vi "DllFxpAddSub_Fxp.vi"(6 "cin/nbin":bool, 8 "load":bool=TRUE, 9 "is sub":bool, 10 "y":fxp<+,32,32>, 11 "x":fxp<+,32,32>) -> (2 "cout/nbout/overflow":bool, 3 "s":fxp<+,32,32>)   [LabVIEW 2017]
uses:
  <vilib>/rvi/FXPMathLib/sim/FxpSim.dll
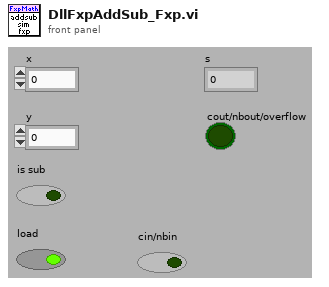
[diagram p1: front panel]
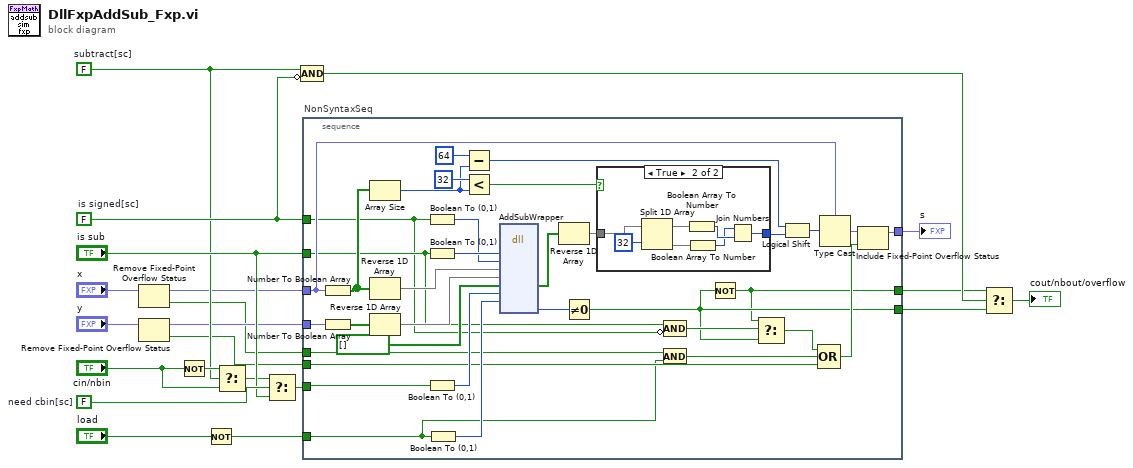
[diagram p0: block diagram]
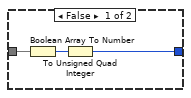
[diagram p2: hidden frame]
diagram:
  w11 = FALSE  # subtract[sc]
  w12 = FALSE  # is signed[sc]
  w21 = FALSE  # need cbin[sc]
  n1 = Remove Fixed-Point Overflow Status(3:"x") -> (0:w3:bool, 1:w6:fxp<+,32,32>)
  n2 = Remove Fixed-Point Overflow Status(3:"y") -> (0:w2:bool, 1:w4:fxp<+,32,32>)
  n3 = Not(x="cin/nbin") -> (.not. x?=w16:bool)
  n4 = Not(x="load") -> (.not. x?=w9:bool)
  n5 = Select(t=w16, s=w11, f="cin/nbin") -> (s? t:f=w17:bool)
  n6 = Select(t=w17, s=w21, f="is sub") -> (s? t:f=w20:bool)
  n7 = Compound Arithmetic op=AND(w11, invert w12) -> (w10:bool)
  n8 = stacked-sequence "NonSyntaxSeq" {
    tunnel: [w24] -> w14
    tunnel: "is sub" -> [w27]
    tunnel: w20 -> [w54]
    tunnel: w9 -> [w30]
    tunnel: w12 -> [w26]
    tunnel: w6 -> [w35]
    tunnel: w4 -> [w42]
    tunnel: [w33] -> w8
    tunnel: w3 -> [w29]
    tunnel: w2 -> [w31]
    tunnel: [w23] -> w1
    frame #0 {
      n9 = Number To Boolean Array(number=w35) -> (Boolean array=w43:bool[])
      n10 = Number To Boolean Array(number=w42) -> (Boolean array=w41:bool[])
      n11 = Array Size(array=w43) -> (size(s)=w40:i32)
      n12 = Reverse 1D Array(array=w43) -> (reversed array=w44:bool[])
      n13 = Reverse 1D Array(array=w41) -> (reversed array=w45:bool[])
      n14 = Boolean To (0,1)(Boolean=w26) -> (0, 1=w55:i16)
      n15 = Boolean To (0,1)(Boolean=w27) -> (0, 1=w56:i16)
      n16 = Boolean To (0,1)(Boolean=w54) -> (0, 1=w50:i16)
      n17 = Boolean To (0,1)(Boolean=w30) -> (0, 1=w51:i16)
      n18 = Subtract(x=64, y=w40) -> (x-y=w37:i32)
      n19 = Less?(x=32, y=w40) -> (x < y?=w46:bool)
      n20 = dll-call lib="e:/penguin/lvdist/win32/export/17.0/17.0.1f1/dist/vi.lib/rvi/FXPMathLib/sim/FxpSim.dll" fn="AddSubWrapper"("isSub"=w56, "isSigned"=w55, "xH"=w44, "yH"=w45, "zH"=bool[] [] ("xH"), "CinOrNBin"=w50, "notLoad"=w51) -> ("zH"=w48:bool[], "CoutOrNBoutOrOvfl"=w52:u8)  [unwired: 3 in, 10 out]
      n21 = Reverse 1D Array(array=w48) -> (reversed array=w53:bool[])
      n22 = Not Equal To 0?(x=w52) -> (x != 0?=w24:bool)
      n23 = case shown="True" w46 {
        tunnel: w53 -> [w59 w66]
        tunnel: [w57 w60] -> w38
        frame False {
          n24 = Boolean Array To Number(Boolean array=w59) -> (number=w58:u32)
          n25 = To Unsigned Quad Integer(1:w58) -> (0:w57:u64)
        }
        frame True {
          n26 = Split 1D Array(array=w66, index=32) -> (first subarray=w64:bool[], second subarray=w63:bool[])
          n27 = Boolean Array To Number(Boolean array=w64) -> (number=w62:u32)
          n28 = Boolean Array To Number(Boolean array=w63) -> (number=w61:u32)
          n29 = Join Numbers(hi=w61, lo=w62) -> ((hi.lo)=w60:u64)
        }
      }
      n30 = And(x=w29, y=w30) -> (x .and. y?=w28:bool)
      n31 = Compound Arithmetic op=AND(w27, invert w26) -> (w25:bool)
      n32 = Not(x=w24) -> (.not. x?=w23:bool)
      n33 = Select(t=w23, s=w25, f=w24) -> (s? t:f=w22:bool)
      n34 = Logical Shift(y=w37, x=w38) -> (x << y=w36:u64)
      n35 = Compound Arithmetic op=OR(w22, w28, w31) -> (w32:bool)
      n36 = Type Cast(type=w35, x=w36) -> (*(type *) &x=w34:fxp<+,32,32>)
      n37 = Include Fixed-Point Overflow Status(2:w32, 3:w34) -> (1:w33:fxp<+,32,32>)
    }
  }
  "s" <- w8
  n38 = Select(t=w1, s=w10, f=w14) -> (s? t:f=→"cout/nbout/overflow":bool)
